vi "A2i.vi"() -> ()   [LabVIEW 2020]
doc: "Use this template to simulate the generation and display of data.\nNote: LabVIEW enables automatic error handling by default for VIs you create from this template."
uses:
  Instance           1 27Saved   GenerateDisplay.vit .vi
panel:
  in  "Frequency":dbl(knob) scale=1.0..10000.0
  in  "Amplitude":dbl(knob) scale=0.0..10.0
  out "Waveform Graph":dynamicdata(graph)
  in  "stop":bool
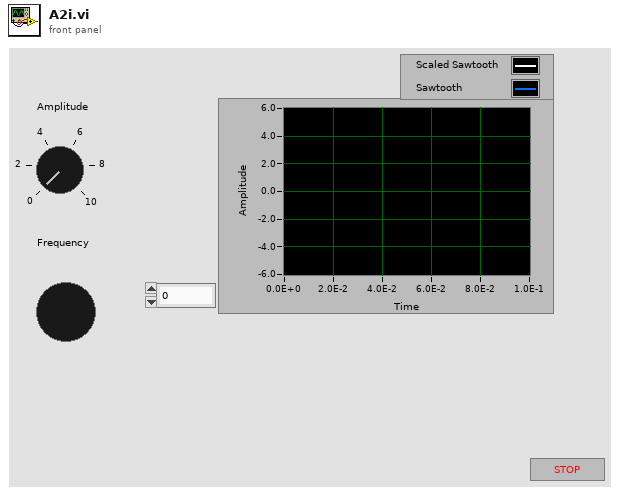
[diagram p1: front panel]
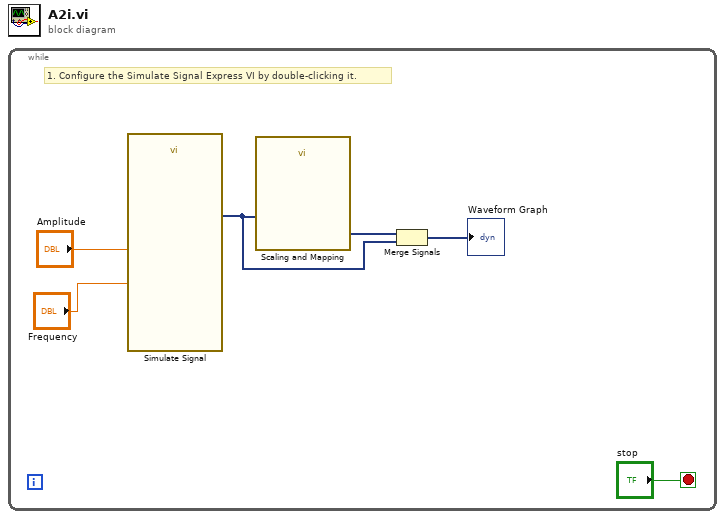
[diagram p0: block diagram]
diagram:
  n1 = while {
    stop <- "stop" stop-if-true
    # "1. Configure the Simulate Signal Express VI by double-clicking it."
    n2 = call "Simulate Signal"("Frequency"="Frequency", "Amplitude"="Amplitude") -> ("Sawtooth"=w2:dynamicdata)  [unwired: 12 in, 1 out]
    n3 = call "Scaling and Mapping"("Signals"=w2) -> ("Scaled Signals"=w4:dynamicdata)  [unwired: 9 in, 1 out]
    n4 = Merge Signals(w4, w2) -> (→"Waveform Graph":dynamicdata)
  }
